vi "Write List of Worksheets.vi"(8 "error in (no error)":errorcluster, 10 "List of Worksheets":string[](array[string]), 11 "Excel Saver in":refnum<class "Excel Saver.lvclass">) -> (0 "error out":errorcluster, 3 "Excel Saver out":refnum<class "Excel Saver.lvclass">)   [LabVIEW 2016, in "Data Saving.lvlib" / "Excel Saver.lvclass"]
uses:
  Excel Saver.lvclass
  Excel Saver.lvclass/Excel Saver.ctl
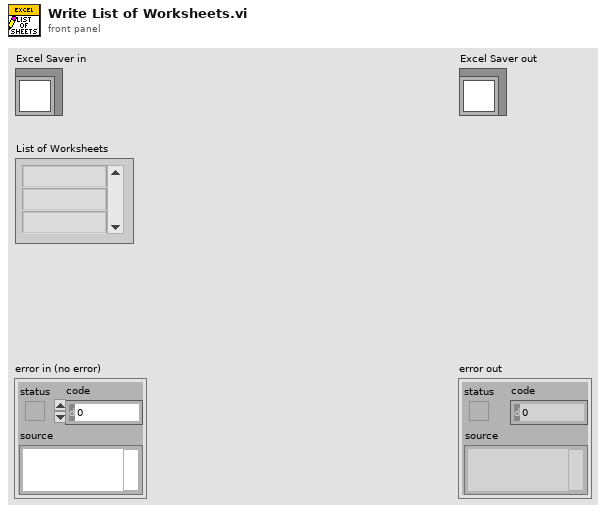
[diagram p1: front panel]
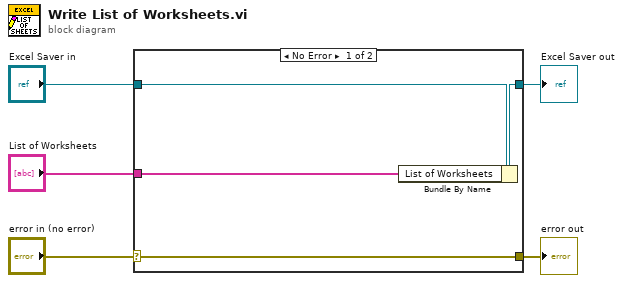
[diagram p0: block diagram]
diagram:
  n1 = case shown="No Error" "error in (no error)" {
    selector: "error in (no error)" -> [w9 w10]
    tunnel: [w9 w10] -> w4
    tunnel: [w7 w11] -> w2
    tunnel: "Excel Saver in" -> [w8 w11]
    tunnel: "List of Worksheets" -> [w6 _]
    frame No Error {
      n2 = Bundle By Name(cluster=w8, "List of Worksheets"=w6) -> (w7:refnum<class "Excel Saver.lvclass">)
    }
    frame Error {
    }
  }
  "error out" <- w4
  "Excel Saver out" <- w2
